vi "Test Clahe Image.vi"(8 "error in (no error)":errorcluster, 11 "Test Case In":refnum<class "01_Image.lvclass">) -> (0 "error out":errorcluster, 3 "Test Case Out":refnum<class "01_Image.lvclass">)   [LabVIEW 2020, in "test.lvlib" / "01_Image.lvclass"]
uses:
  01_Image.lvclass
  C:/Program Files (x86)/National Instruments/LabVIEW 2020/vi.lib/Astemes/LUnit/Test Case.lvclass
  image/CLAHE/CLAHE.lvclass/CLAHE.ctl
  <vilib>/Astemes/LUnit/Test Case.lvclass/Test Case.ctl
  image/New Image (Greyscale Array).vi
  image/New Image (Greyscale Preallocated).vi
  image/CLAHE/Apply (Greyscale Image).vi
  4993e8ee-a06a-463a-9684-69129f64d5ce.vi
  image/New Image (Greyscale Preallocated).vi/6598b9e0-8a08-46f5-91fd-ca1b87217137.vi
  <vilib>/Astemes/LUnit/Core/LUnit Test Case/Private/Append Pass Result.vi
  <vilib>/Astemes/LUnit/Core/LUnit Test Case/Private/Append Fail Result.vi
  4993e8ee-a06a-463a-9684-69129f64d5ce.vi/9c5d11cd-9439-4240-a1ee-d9baace9c924.vi
  <vilib>/Astemes/LUnit/Core/LUnit Test Case/Private/Run In UI.vi
  <vilib>/Utility/error.llb/Clear Errors.vi
  <vilib>/Utility/error.llb/Error Cluster From Error Code.vi
  image/CLAHE/CLAHE.lvclass
  01_Image.lvclass/01_Image.ctl
  image/image.lvlib
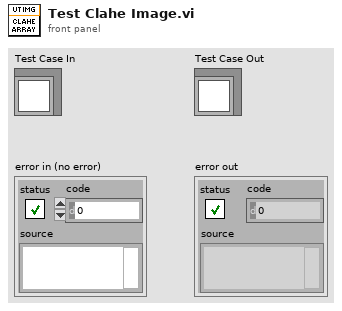
[diagram p1: front panel]
types:
  T1 = typedef "image.lvlib/Greyscale Image.ctl" = refnum<data-value>
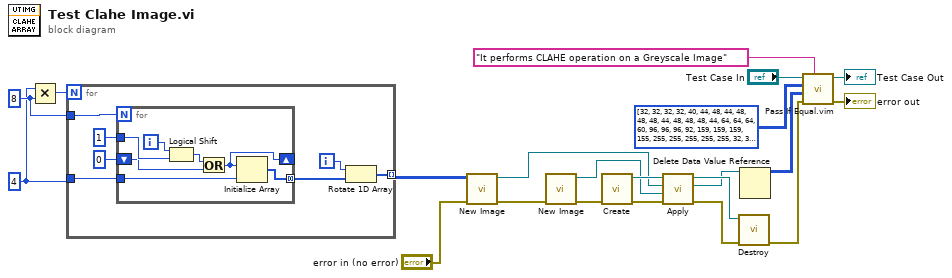
[diagram p0: block diagram]
diagram:
  w9 = 4 ("dimension size")
  w11 = 8
  n1 = Multiply(x=w9, y=w11) -> (x*y=w10:i32)
  n2 = for {
    N: w10 -> [_]
    tunnel: [w26] -> w6 mode=indexing
    tunnel: w11 -> [w25]
    tunnel: w9 -> [w24]
    i -> [w27]
    n3 = for {
      N: w25 -> [_]
      tunnel: [w33] -> w28 mode=concatenating
      tunnel: w24 -> [w32]
      tunnel: u8 1 ("x") -> [w31]
      shift-right: [w29] -> _
      shift-left: u8 0 -> [w30]
      i -> [w35]
      n4 = Logical Shift(y=w35, x=w31) -> (x << y=w34:u8)
      n5 = Or(x=w34, y=w30) -> (x .or. y?=w29:u8)
      n6 = Initialize Array(w29, w32) -> (w33:u8[])
    }
    n7 = Rotate 1D Array(1:w28, 2:w27) -> (0:w26:u8[])
  }
  n8 = call-poly "New Image.vi"("error in (no error)"="error in (no error)", "U8 Greyscale Data"=w6) -> ("error out"=w4:errorcluster, "Greyscale Image"=w3:T1)  [unwired: 8 in]
  n9 = call-poly "New Image.vi"("error in (no error)"=w4) -> ("error out"=w15:errorcluster, "Greyscale Image"=w16:T1)  [unwired: 9 in]
  n10 = call "Create.vi"("error in (no error)"=w15) -> ("error out"=w14:errorcluster, "CLAHE"=w18:refnum<class "CLAHE.lvclass">)  [unwired: 9 in]
  n11 = call-poly "Apply.vi"("error in (no error)"=w14, "Destination Image in"=w16, "Greyscale Image in"=w3, "CLAHE in"=w18) -> ("error out"=w13:errorcluster, "Destination Image"=w8:T1, "CLAHE"=w17:refnum<class "CLAHE.lvclass">)  [unwired: 5 in]
  n12 = call "Destroy.vi"("error in (no error)"=w13, "CLAHE"=w17) -> ("error out"=w12:errorcluster)  [unwired: 9 in]
  n13 = Delete Data Value Reference(data value reference=w8) -> (data value=w2:u8[][])  [unwired: 1 in, 1 out]
  n14 = call "Pass If Equal.vim"("Description"="It performs CLAHE operation on a Greyscale Image", "error in (no error)"=w12, "Actual"=w2, "Expected"=u8[][] [[32, 32, 32, 32, 40, 44, 48, 44, 48, 48, 48, 44, 48, 48, 48, 44, 64, 64, 64, 60, 96, 96, 96, 92, 159, 159, 159, 155, 255, 255, 255, 255], [255, 32, 32, 32, 32, 44, 48, 44, 40, 48, 48, 44, 40, 48, 48, 44, 40, 64, 64, 60, 56, 96, 96, 92, 88, 159, 159, 155, 151, 255, 255, 255], [255, 255, 32, 32, 32, 32, 48, 44, 40, 36, 48, 44, 40, 36, 48, 44, 40, 36, 64, 60, 56, 52, 96, 92, 88, 84, 159, 155, 151, 147, 255, 255], [255, 255, 255, 29, 30, 31, 32, 42, 40, 38, 36, 45, 42, 39, 36, 45, 42, 39, 36, 61, 58, 55, 52, 93, 90, 87, 84, 156, 153, 150, 147, 255], [255, 255, 255, 255, 28, 30, 32, 30, 40, 40, 40, 36, 44, 42, 40, 36, 44, 42, 40, 36, 60, 58, 56, 52, 92, 90, 88, 84, 155, 153, 151, 151], [143, 255, 255, 255, 255, 29, 32, 31, 30, 42, 44, 40, 36, 45, 44, 40, 36, 45, 44, 40, 36, 61, 60, 56, 52, 93, 92, 88, 84, 156, 155, 155], [143, 143, 255, 255, 255, 255, 32, 32, 32, 32, 48, 44, 40, 36, 48, 44, 40, 36, 48, 44, 40, 36, 64, 60, 56, 52, 96, 92, 88, 84, 159, 159], [147, 147, 147, 255, 255, 255, 255, 29, 30, 31, 32, 42, 40, 38, 36, 45, 42, 39, 36, 45, 42, 39, 36, 61, 58, 55, 52, 93, 90, 87, 84, 159], [151, 151, 151, 149, 255, 255, 255, 255, 28, 30, 32, 30, 40, 40, 40, 36, 44, 42, 40, 36, 44, 42, 40, 36, 60, 58, 56, 52, 92, 90, 88, 88], [76, 155, 155, 152, 149, 255, 255, 255, 255, 29, 32, 31, 30, 42, 44, 40, 36, 45, 44, 40, 36, 45, 44, 40, 36, 61, 60, 56, 52, 93, 92, 92], [80, 80, 159, 155, 151, 147, 255, 255, 255, 255, 32, 32, 32, 32, 48, 44, 40, 36, 48, 44, 40, 36, 48, 44, 40, 36, 64, 60, 56, 52, 96, 96], [84, 84, 84, 156, 153, 150, 147, 255, 255, 255, 255, 29, 30, 31, 32, 42, 40, 38, 36, 45, 42, 39, 36, 45, 42, 39, 36, 61, 58, 55, 52, 96], [88, 88, 88, 84, 155, 153, 151, 149, 255, 255, 255, 255, 28, 30, 32, 30, 40, 40, 40, 36, 44, 42, 40, 36, 44, 42, 40, 36, 60, 58, 56, 56], [44, 92, 92, 88, 84, 156, 155, 152, 149, 255, 255, 255, 255, 29, 32, 31, 30, 42, 44, 40, 36, 45, 44, 40, 36, 45, 44, 40, 36, 61, 60, 60], [48, 48, 96, 92, 88, 84, 159, 155, 151, 147, 255, 255, 255, 255, 32, 32, 32, 32, 48, 44, 40, 36, 48, 44, 40, 36, 48, 44, 40, 36, 64, 64], [52, 52, 52, 93, 90, 87, 84, 156, 153, 150, 147, 255, 255, 255, 255, 29, 30, 31, 32, 42, 40, 38, 36, 45, 42, 39, 36, 45, 42, 39, 36, 64], [56, 56, 56, 52, 92, 90, 88, 84, 155, 153, 151, 149, 255, 255, 255, 255, 28, 30, 32, 30, 40, 40, 40, 36, 44, 42, 40, 36, 44, 42, 40, 40], [28, 60, 60, 56, 52, 93, 92, 88, 84, 156, 155, 152, 149, 255, 255, 255, 255, 29, 32, 31, 30, 42, 44, 40, 36, 45, 44, 40, 36, 45, 44, 44], [32, 32, 64, 60, 56, 52, 96, 92, 88, 84, 159, 155, 151, 147, 255, 255, 255, 255, 32, 32, 32, 32, 48, 44, 40, 36, 48, 44, 40, 36, 48, 48], [36, 36, 36, 61, 58, 55, 52, 93, 90, 87, 84, 156, 153, 150, 147, 255, 255, 255, 255, 29, 30, 31, 32, 42, 40, 38, 36, 45, 42, 39, 36, 48], [40, 40, 40, 36, 60, 58, 56, 52, 92, 90, 88, 84, 155, 153, 151, 149, 255, 255, 255, 255, 28, 30, 32, 30, 40, 40, 40, 36, 44, 42, 40, 40], [28, 44, 44, 40, 36, 61, 60, 56, 52, 93, 92, 88, 84, 156, 155, 152, 149, 255, 255, 255, 255, 29, 32, 31, 30, 42, 44, 40, 36, 45, 44, 44], [32, 32, 48, 44, 40, 36, 64, 60, 56, 52, 96, 92, 88, 84, 159, 155, 151, 147, 255, 255, 255, 255, 32, 32, 32, 32, 48, 44, 40, 36, 48, 48], [36, 36, 36, 45, 42, 39, 36, 61, 58, 55, 52, 93, 90, 87, 84, 156, 153, 150, 147, 255, 255, 255, 255, 29, 30, 31, 32, 42, 40, 38, 36, 48], [40, 40, 40, 36, 44, 42, 40, 36, 60, 58, 56, 52, 92, 90, 88, 84, 155, 153, 151, 149, 255, 255, 255, 255, 28, 30, 32, 30, 40, 40, 40, 40], [28, 44, 44, 40, 36, 45, 44, 40, 36, 61, 60, 56, 52, 93, 92, 88, 84, 156, 155, 152, 149, 255, 255, 255, 255, 29, 32, 31, 30, 42, 44, 44], [32, 32, 48, 44, 40, 36, 48, 44, 40, 36, 64, 60, 56, 52, 96, 92, 88, 84, 159, 155, 151, 147, 255, 255, 255, 255, 32, 32, 32, 32, 48, 48], [36, 36, 36, 45, 42, 39, 36, 45, 42, 39, 36, 61, 58, 55, 52, 93, 90, 87, 84, 156, 153, 150, 147, 255, 255, 255, 255, 29, 30, 31, 32, 44], [40, 40, 40, 36, 44, 42, 40, 36, 44, 42, 40, 36, 60, 58, 56, 52, 92, 90, 88, 84, 155, 153, 151, 149, 255, 255, 255, 255, 28, 30, 32, 32], [28, 44, 44, 40, 36, 45, 44, 40, 36, 45, 44, 40, 36, 61, 60, 56, 52, 93, 92, 88, 84, 156, 155, 152, 149, 255, 255, 255, 255, 29, 32, 32], [32, 32, 48, 44, 40, 36, 48, 44, 40, 36, 48, 44, 40, 36, 64, 60, 56, 52, 96, 92, 88, 84, 159, 155, 151, 147, 255, 255, 255, 255, 32, 32], [32, 32, 32, 44, 40, 36, 32, 44, 40, 36, 32, 44, 40, 36, 32, 60, 56, 52, 48, 92, 88, 84, 80, 155, 151, 147, 143, 255, 255, 255, 255, 32]] ("data value"), "LUnit Test Case In"="Test Case In") -> ("error out"=→"error out":errorcluster, "LUnit Test Case Out"=→"Test Case Out":refnum<class "01_Image.lvclass">)  [unwired: 5 in]
